vi "ep_Power Spectrum.vi"(0 "phase voltage spectra (5Hz step)":T2(array[cluster]), 5 "current spectra (5Hz step)":T2(array[cluster]), 9 "system info in":refnum<class "EP System Info.lvclass">, 11 "error in (no error)":errorcluster) -> (2 "fundamental active power P1 (W)":dbl[](array[numeric]), 3 "cosine":dbl[](array[numeric]), 4 "active power P (W)":dbl[](array[numeric]), 6 "reactive power Q (VAr)":dbl[](array[numeric]), 8 "apparent power S (VA)":dbl[](array[numeric]), 10 "system info out":refnum<class "EP System Info.lvclass">, 13 "power factor PF":dbl[](array[numeric]), 14 "fundamental reactive power Q1 (VAr)":dbl[](array[numeric]), 15 "error out":errorcluster)   [LabVIEW 2013, in "NI_EP_Power Quality.lvlib"]
doc: "This VI calculates power spectra."
uses:
  <vilib>/addons/Electrical Power/PQ/NI_EP_Power Quality.lvlib
  <vilib>/addons/Electrical Power/PQ/Common/Controls/ep_AI Data Channel.ctl
  <vilib>/addons/Electrical Power/PQ/Common/Classes/System Info/EP System Info.lvclass
  <vilib>/addons/Electrical Power/Power Measurement/NI_EP_Power Measurement.lvlib
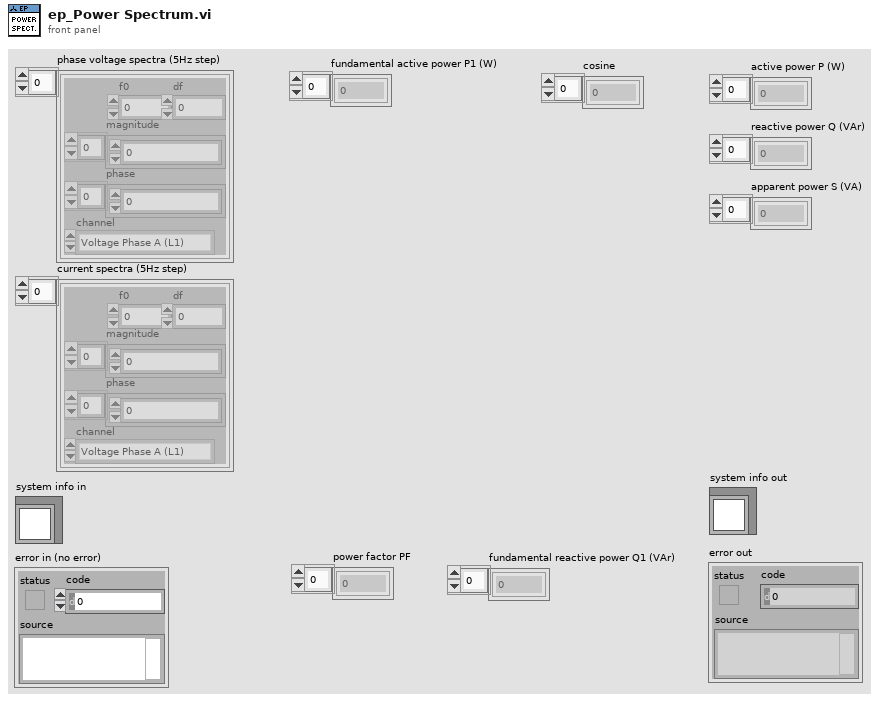
[diagram p1: front panel]
types:
  T1 = typedef "NI_EP_Power Quality.lvlib/ep_AI Data Channel.ctl" = enum16{"Voltage Phase A (L1)", "Voltage Phase B (L2)", "Voltage Phase C (L3)", "Voltage Phase N (Neutral)", "Current Phase A (L1)", "Current Phase B (L2)", "Current Phase C (L3)", "Current Phase N (Neutral)"}
  T2 = cluster{"f0":dbl, "df":dbl, "magnitude":dbl[], "phase":dbl[], "channel":T1}[]
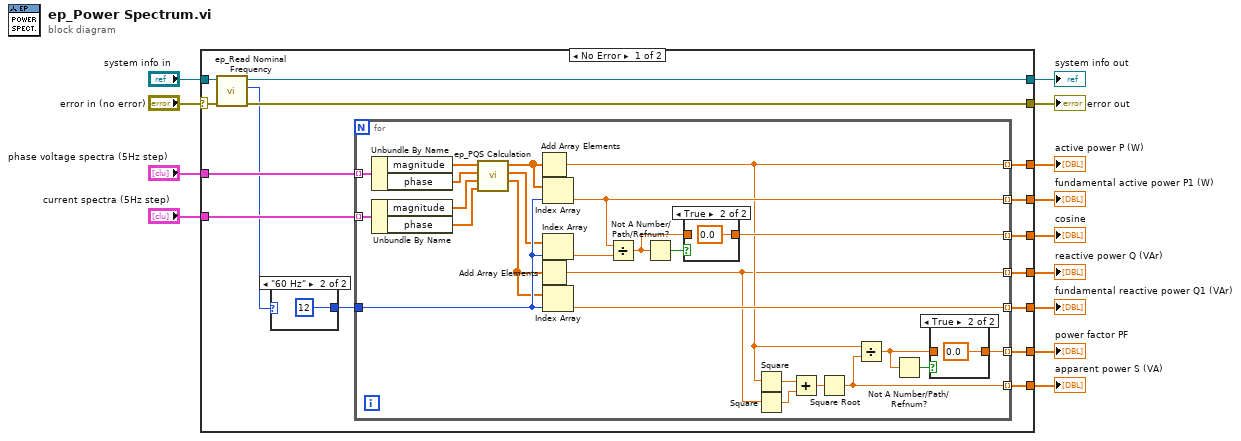
[diagram p0: block diagram]
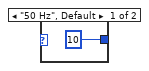
[diagram p2: hidden frame]
diagram:
  n1 = case shown="No Error" "error in (no error)" {
    selector: "error in (no error)" -> [w25 w60]
    tunnel: "current spectra (5Hz step)" -> [w28 _]
    tunnel: "phase voltage spectra (5Hz step)" -> [w27 _]
    tunnel: [w24 w60] -> w8
    tunnel: "system info in" -> [w26 _]
    tunnel: [w23 _] -> w9
    tunnel: [w20 _] -> w7
    tunnel: [w19 _] -> w6
    tunnel: [w18 _] -> w5
    tunnel: [w17 _] -> w4
    tunnel: [w16 _] -> w2
    tunnel: [w15 _] -> w3
    tunnel: [w14 _] -> w1
    frame No Error {
      n2 = call <vilib>:"ep_Read Nominal Frequency.vi"("error in (no error)"=w25, "system info in"=w26) -> ("error out"=w24:errorcluster, "nominal frequency"=w22:enum16{"50 Hz", "60 Hz"}, "system info out"=w23:refnum<class "EP System Info.lvclass">)  [unwired: 6 in, 1 out]
      n3 = case shown="\"60 Hz\"" w22 {
        tunnel: [10 12] -> w21
        frame "50 Hz", Default {
        }
        frame "60 Hz" {
        }
      }
      n4 = for {
        tunnel: w27 -> [w55] mode=indexing
        tunnel: w28 -> [w35] mode=indexing
        tunnel: w21 -> [w49]
        tunnel: [w44] -> w20 mode=indexing
        tunnel: [w53] -> w19 mode=indexing
        tunnel: [w50] -> w18 mode=indexing
        tunnel: [w43] -> w17 mode=indexing
        tunnel: [w46] -> w16 mode=indexing
        tunnel: [w45] -> w15 mode=indexing
        tunnel: [w39] -> w14 mode=indexing
        n5 = Unbundle By Name(w55) -> ("magnitude"=w34:dbl[], "phase"=w33:dbl[])
        n6 = Unbundle By Name(w35) -> ("magnitude"=w32:dbl[], "phase"=w31:dbl[])
        n7 = call <vilib>:"ep_PQS Calculation.vi"("I phase"=w31, "I magnitute"=w32, "U phase"=w33, "U magnitute"=w34) -> ("Q"=w36:dbl[], "S"=w37:dbl[], "P"=w38:dbl[])  [unwired: 5 in]
        n8 = Add Array Elements(numeric array=w38) -> (sum=w44:dbl)
        n9 = Add Array Elements(numeric array=w36) -> (sum=w43:dbl)
        n10 = Index Array(array=w38, index=w49) -> (element=w53:dbl)
        n11 = Index Array(array=w37, index=w49) -> (element=w54:dbl)
        n12 = Index Array(array=w36, index=w49) -> (element=w45:dbl)
        n13 = Divide(x=w53, y=w54) -> (x/y=w51:dbl)
        n14 = Not A Number/Path/Refnum?(number/path/refnum=w51) -> (NaN/Path/Refnum?=w52:bool)
        n15 = case shown="True" w52 {
          tunnel: w51 -> [w58 _]
          tunnel: [w58 0.0] -> w50
          frame False {
          }
          frame True {
          }
        }
        n16 = Square(x=w44) -> (x^2=w42:dbl)
        n17 = Square(x=w43) -> (x^2=w41:dbl)
        n18 = Add(x=w42, y=w41) -> (x+y=w40:dbl)
        n19 = Square Root(x=w40) -> (sqrt(x)=w39:dbl)
        n20 = Divide(x=w44, y=w39) -> (x/y=w47:dbl)
        n21 = Not A Number/Path/Refnum?(number/path/refnum=w47) -> (NaN/Path/Refnum?=w48:bool)
        n22 = case shown="True" w48 {
          tunnel: w47 -> [w56 _]
          tunnel: [w56 0.0] -> w46
          frame False {
          }
          frame True {
          }
        }
      }
    }
    frame Error {
    }
  }
  "error out" <- w8
  "system info out" <- w9
  "active power P (W)" <- w7
  "fundamental active power P1 (W)" <- w6
  "cosine" <- w5
  "apparent power S (VA)" <- w1
  "reactive power Q (VAr)" <- w4
  "fundamental reactive power Q1 (VAr)" <- w3
  "power factor PF" <- w2
